vi "Filter Error Codes (Scalar)__jki_lib_error_handling -- VI Tester.vi"(4 "upstream error (optional)":errorcluster, 8 "error in":errorcluster, 10 "error code to filter":i32) -> (0 "error out":errorcluster, 1 "error filtered?":bool, 2 "filtered error details":T1)   [LabVIEW 2013]
uses:
  Filtered Error Details - Cluster__jki_lib_error_handling -- VI Tester.ctl
panel:
  # "Copyright © 2007 James Kring, Inc. All rights reserved.\n\nAuthor: Jim Kring <jim.kring@jameskring.com>\n\nThis library is provided \"AS IS\" , WITHOUT WARRANTIES OR \nCONDITIONS OF ANY KIND, either express or implied.\n\nJames Kring, Inc. -- http://www.jameskring.com"
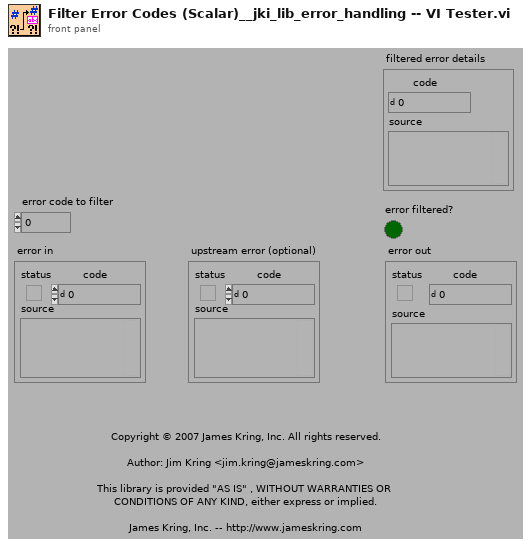
[diagram p1: front panel]
types:
  T1 = typedef "Filtered Error Details - Cluster__jki_lib_error_handling -- VI Tester.ctl" = cluster{"code":i32, "source":string}
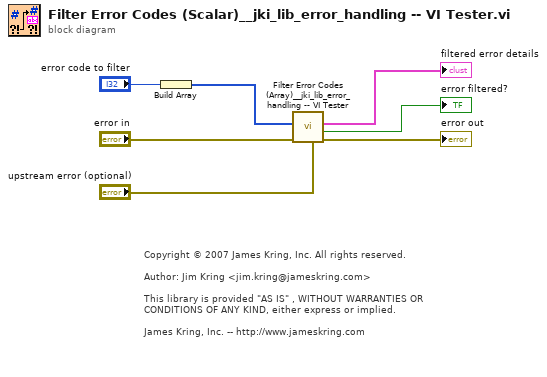
[diagram p0: block diagram]
diagram:
  # "Copyright © 2007 James Kring, Inc. All rights reserved.\n\nAuthor: Jim Kring <jim.kring@jameskring.com>\n\nThis library is provided \"AS IS\" , WITHOUT WARRANTIES OR \nCONDITIONS OF ANY KIND, either express or implied.\n\nJames Kring, Inc. -- http://www.jameskring.com"
  n1 = Build Array("error code to filter") -> (w4:i32[])
  n2 = call "Filter Error Codes (Array)__jki_lib_error_handling -- VI Tester.vi"("upstream error (optional)"="upstream error (optional)", "error in"="error in", "error codes to filter"=w4) -> ("error out"=→"error out":errorcluster, "error filtered?"=→"error filtered?":bool, "filtered error details"=→"filtered error details":T1)  [unwired: 6 in]
